vi "MH_T2 Read Acq Q_RawTimes.vi"() -> ()   [LabVIEW 2019]
uses:
  <userlib>/MultiHarp150/T2Lib/MH_T2QMessage.ctl
  <userlib>/MultiHarp150/T2Lib/MH_T2DeltaQMessage.ctl
  <vilib>/Analysis/NI_AALBase.lvlib
panel:
  out "valeur min":u64
  out "valeur max":u64
  out "Tableau":u64[][](array[numeric])
  out "Histogram: h(x)":i32[][](array[numeric])
  in  "Graphsamples":i32
  out "Graphe XY 2":T1(graph)
  in  "intervals":i32=10
  in  "Delta":bool
  in  "Graphe":bool
  out "Graphe XY":cluster{u64[], u64[]}[](graph)
  out "Photons":u64[][](array[numeric])
  out "taille(s)":i32[](array[numeric])
  out "Counters out":u32[](array[numeric])
  in  "TraceSize":u64
  in  "Bin size(ps)":u64
  in  "Tracelenght(s)":u64=16
  out "Done":bool
  out "TotalRec":i32
  out "TotalTime":u32
  in  "stop":bool
  out "sortie d'erreur":errorcluster caption="ErrorOut"
  out "RollOver":bool
  in  "Save Data":bool
  in  "StopCh":u32=2
  in  "StartCh":u32=1
  out "DeltaT":u32[](array[numeric])
  out "nActual":i32[](array[numeric])
  out "En Attente":i32[](array[numeric])
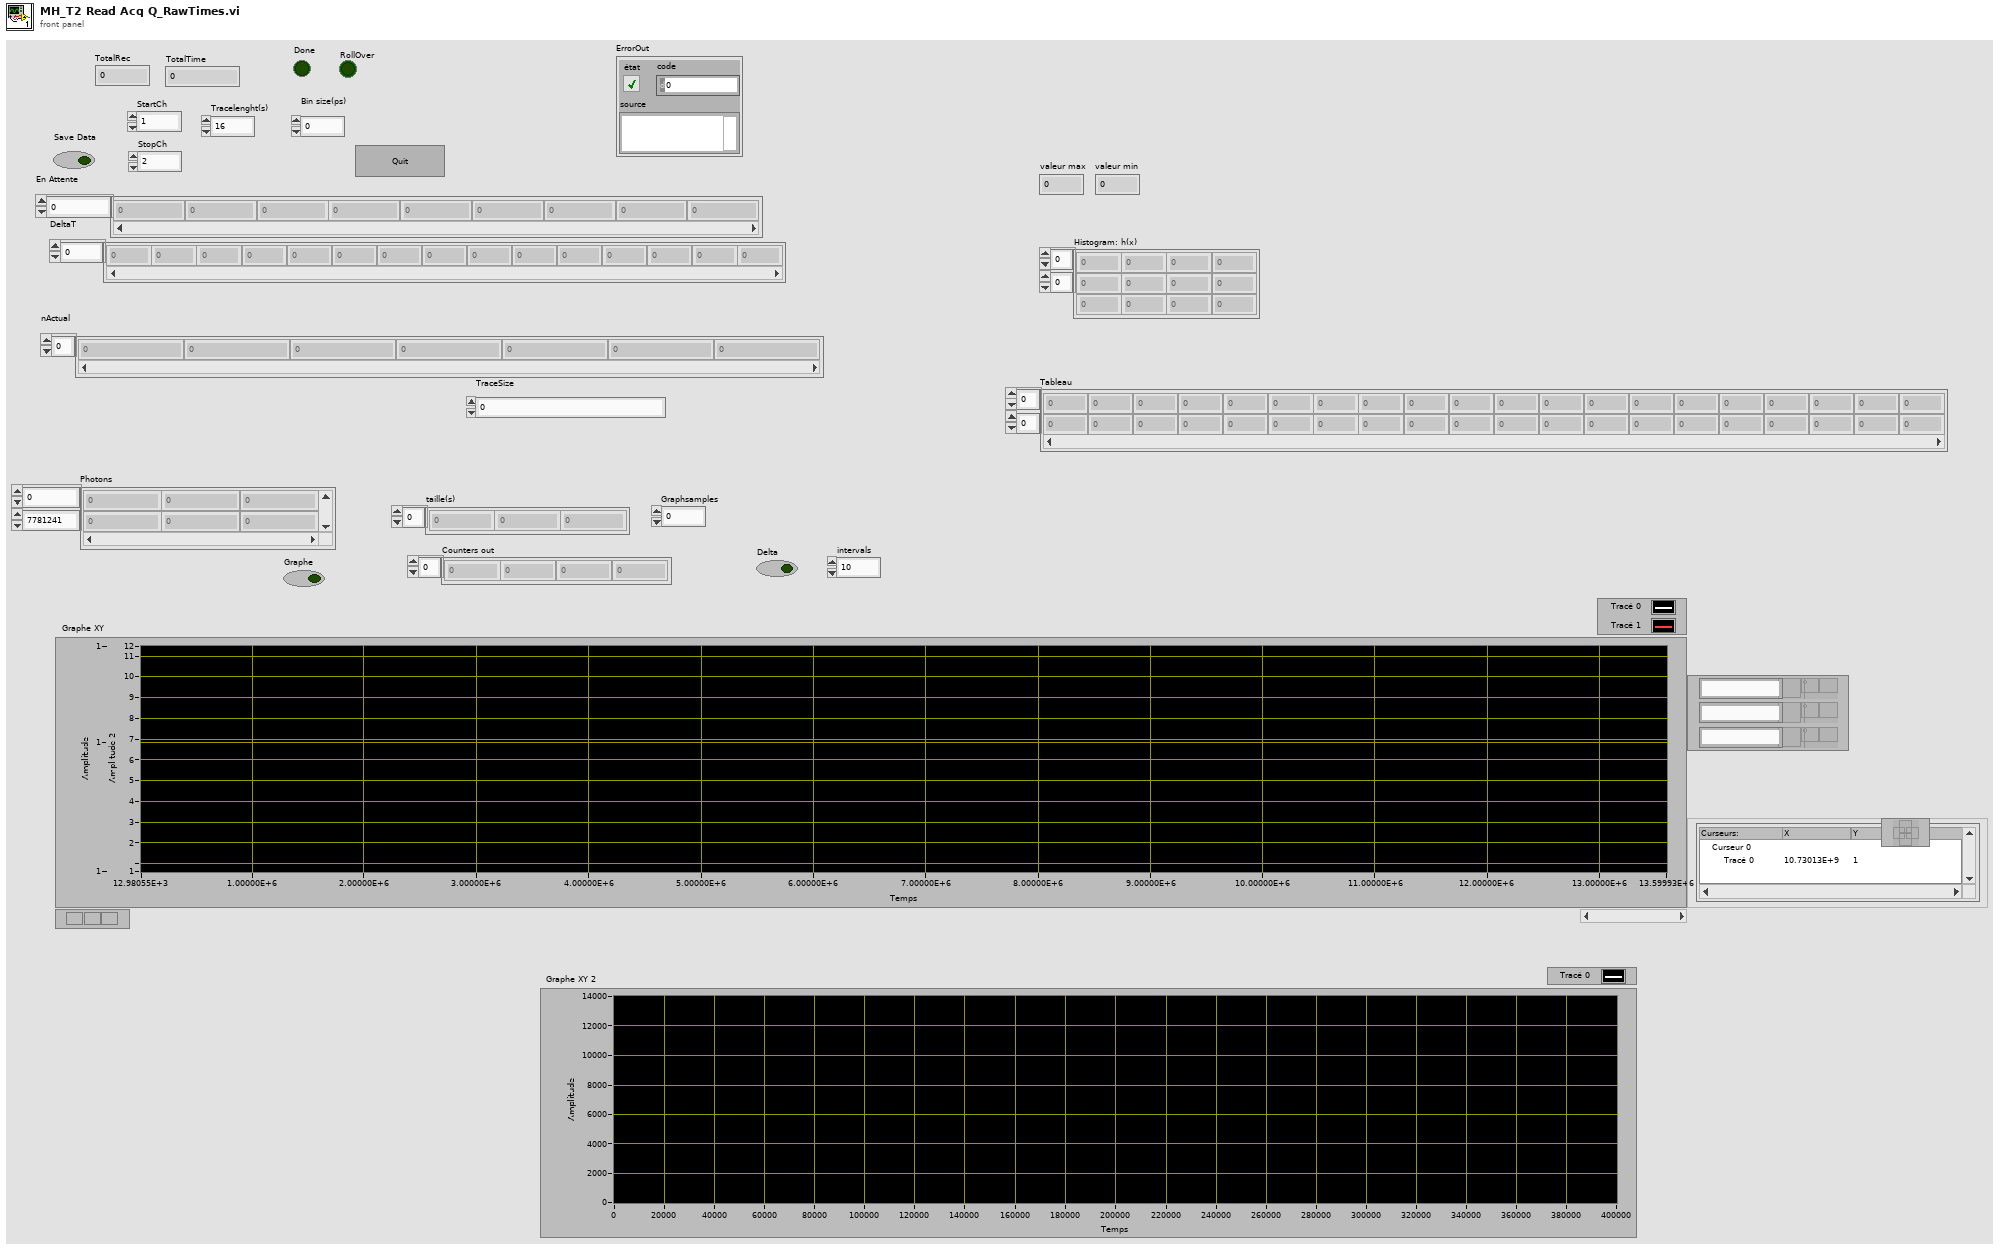
[diagram p1: front panel]
types:
  T1 = cluster{"X Values":dbl[], "Histogram: h(x)":i32[]}[]
  T2 = typedef "MH_T2DeltaQMessage.ctl" = cluster{"Message":string, "buffer":i32[], "Code":i32, "nactual":i32}
  T3 = typedef "MH_T2QMessage.ctl" = cluster{"Message":string, "buffer":u32[], "Code":i32, "nactual":i32}
  T4 = cluster{"X Values":dbl[], "Histogram: h(x)":i32[]}
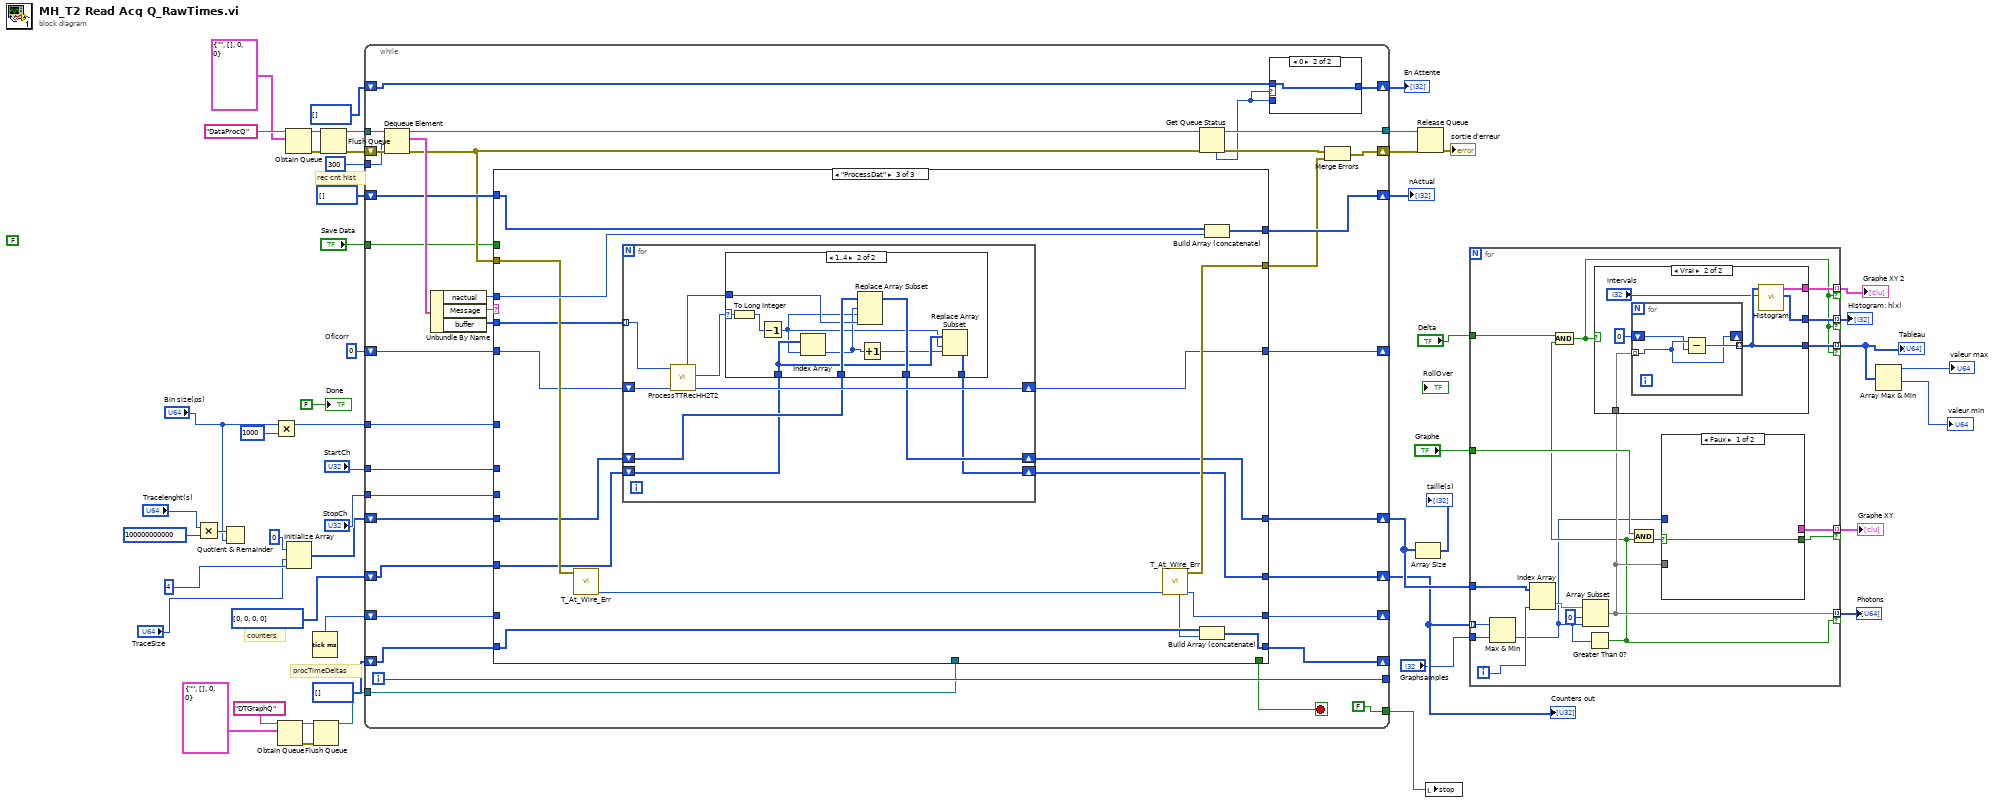
[diagram p0: block diagram]
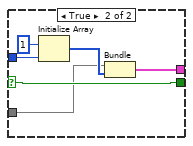
[diagram p3: hidden frame]
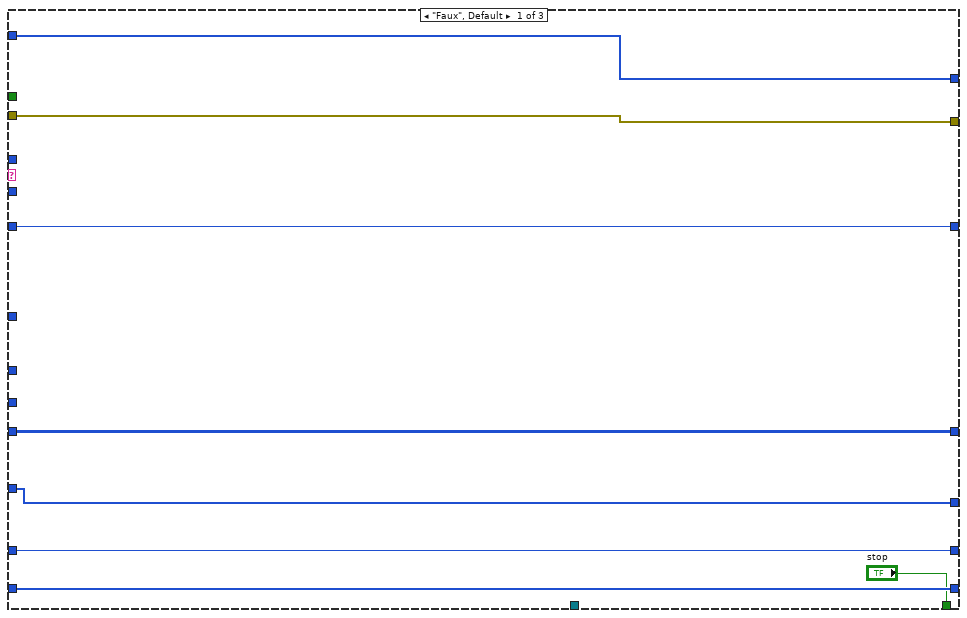
[diagram p4: hidden frame]
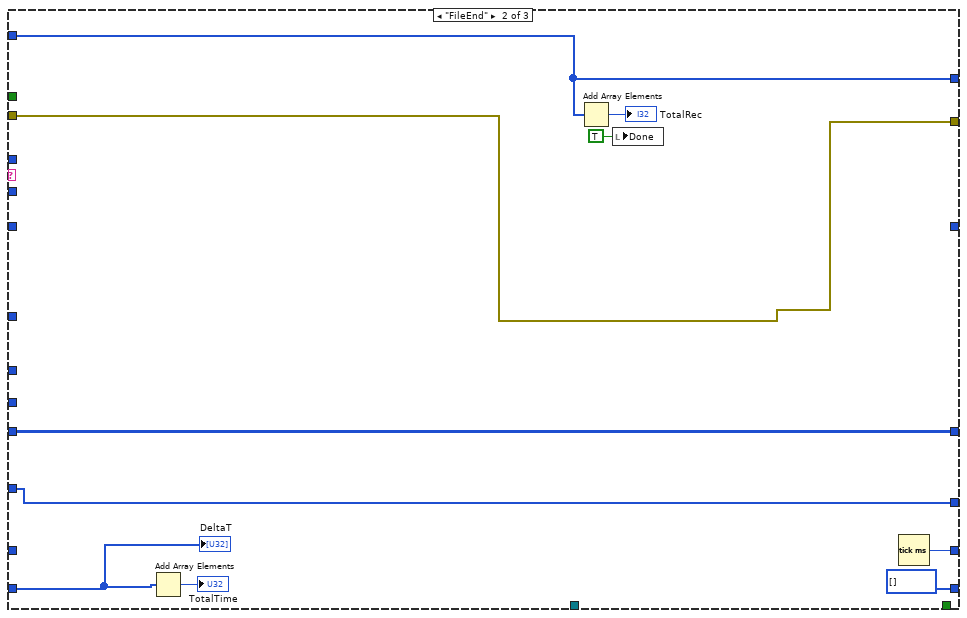
[diagram p5: hidden frame]
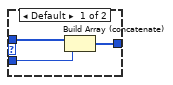
[diagram p7: hidden frame]
diagram:
  (unwired) FALSE
  w49 = u64 0  # Oflcorr
  # "counters"
  # "procTimeDeltas"
  # "rec cnt hist"
  n1 = Multiply(x="Tracelenght(s)", y=u64 100000000000) -> (x*y=w21:u64)
  n2 = Quotient & Remainder(x=w21, y="Bin size(ps)") -> ()  [unwired: 2 out]
  n3 = Multiply(x="Bin size(ps)", y=u64 1000) -> (x*y=w18:u64)
  n4 = Obtain Queue(name (unnamed)="DTGraphQ" ("nom (aucun)"), element data type=T2 {"Message"="", "buffer"=[], "Code"=0, "nactual"=0} ("ClassQueue")) -> (queue out=w27:refnum<queue>, error out=w28:errorcluster)  [unwired: 3 in, 1 out]
  n5 = Obtain Queue(name (unnamed)="DataProcQ" ("nom (aucun)"), element data type=T3 {"Message"="", "buffer"=[], "Code"=0, "nactual"=0} ("ClassQueue")) -> (queue out=w32:refnum<queue>, error out=w29:errorcluster)  [unwired: 3 in, 1 out]
  n6 = Initialize Array(u64 0 ("truetime"), "TraceSize", 4 ("taille de la dimension")) -> (w24:u64[][])
  n7 = Tick Count (ms)() -> (millisecond timer value=w45:u32)
  n8 = Flush Queue(queue=w27, error in (no error)=w28) -> (queue out=w34:refnum<queue>)  [unwired: 2 out]
  n9 = Flush Queue(queue=w32, error in (no error)=w29) -> (queue out=w31:refnum<queue>, error out=w30:errorcluster)  [unwired: 1 out]
  n10 = while {
    tunnel: w31 -> [w86]
    shift-right: [w67] -> w48
    shift-left: w30 -> [w87]
    shift-right: [w84] -> _
    shift-left: w49 -> [w85]
    tunnel: [w81] -> _
    tunnel: [w77] -> w47
    shift-right: [w75] -> _
    shift-left: w45 -> [w76]
    shift-right: [w73] -> _
    shift-left: u32[] [] ("DeltaT") -> [w74]
    shift-right: [w71] -> w42
    shift-left: i32[] [] ("DeltaT") -> [w72]
    shift-right: [w70] -> w46
    shift-left: i32[] [] ("DeltaT") -> [w69]
    tunnel: "Save Data" -> [w66]
    shift-right: [w63] -> w12
    shift-left: w24 -> [w65]
    tunnel: "StopCh" -> [w64]
    tunnel: 300 ("timeout en ms (-1)") -> [w62]
    tunnel: w34 -> [w60]
    tunnel: [FALSE] -> w26
    tunnel: "StartCh" -> [w55]
    tunnel: w18 -> [w54]
    shift-right: [w52] -> w11
    shift-left: i32[] [0, 0, 0, 0] ("DeltaT") -> [w53]
    i -> [w81]
    stop <- w58 stop-if-true
    n11 = Dequeue Element(queue=w86, timeout in ms (-1)=w62, error in (no error)=w87) -> (queue out=w79:refnum<queue>, element=w83:T3, error out=w68:errorcluster)  [unwired: 1 out]
    n12 = Unbundle By Name(w83) -> ("nactual"=w61:i32, "Message"=w80:string, "buffer"=w82:u32[])
    n13 = case shown="\"ProcessDat\"" w80 {
      tunnel: w85 -> [w95 _ w111]
      tunnel: [w95 _ w110] -> w84
      tunnel: w82 -> [_ _ w112]
      tunnel: w76 -> [w94 _ _]
      tunnel: [w93 u32[] [] ("DeltaT") w115] -> w73
      tunnel: [w94 w104 w116] -> w75
      tunnel: w74 -> [w93 w102 w114]
      tunnel: w72 -> [w92 w100 w121]
      tunnel: [w92 w100 w122] -> w71
      tunnel: w68 -> [w90 w97 w119]
      tunnel: w66 -> [_ _ _]
      tunnel: w65 -> [w91 w105 w109]
      tunnel: w64 -> [_ _ _]
      tunnel: [w91 w105 w108] -> w63
      tunnel: w61 -> [_ _ w120]
      tunnel: w60 -> [_ _ _]
      tunnel: [w90 w97 w118] -> w59
      tunnel: ["stop" _ _] -> w58
      tunnel: w55 -> [_ _ _]
      tunnel: w54 -> [_ _ _]
      tunnel: w53 -> [w88 w96 w107]
      tunnel: [w88 w96 w106] -> w52
      frame "Faux", Default {
      }
      frame "FileEnd" {
        n14 = Add Array Elements(numeric array=w102) -> (sum=→"TotalTime":u32)
        n15 = Add Array Elements(numeric array=w100) -> (sum=→"TotalRec":i32)
        n16 = local write "Done"(TRUE ("Done")) -> ()
        n17 = Tick Count (ms)() -> (millisecond timer value=w104:u32)
        "DeltaT" <- w102
      }
      frame "ProcessDat" {
        n18 = call <userlib>:"T_At_Wire_Err.vi"("error in (no error)"=w119) -> ("Clock(ms)"=w117:u32)  [unwired: 8 in, 2 out]
        n19 = for {
          tunnel: w112 -> [w131] mode=indexing
          shift-right: [w129] -> w110
          shift-left: w111 -> [w130]
          shift-right: [w125] -> w108
          shift-left: w109 -> [w126]
          shift-right: [w123] -> w106
          shift-left: w107 -> [w124]
          n20 = call <userlib>:"ProcessTTRecHH2T2.vi"("oflcorr_in"=w130, "rawbits"=w131) -> ("oflcorr_out"=w129:u64, "channel"=w128:u32, "truetime"=w127:u64)  [unwired: 4 in, 3 out]
          n21 = case shown="1..4" w128 {
            selector: w128 -> [_ w137]
            tunnel: w127 -> [_ w141]
            tunnel: w126 -> [w133 w143]
            tunnel: [w133 w142] -> w125
            tunnel: w124 -> [w132 w139]
            tunnel: [w132 w135] -> w123
            frame 0, Default {
            }
            frame 1..4 {
              n22 = To Long Integer(number=w137) -> (32bit integer=w136:i32)
              n23 = Decrement(x=w136) -> (x-1=w134:i32)
              n24 = Index Array(array=w139, index=w134) -> (element=w140:i32)
              n25 = Replace Array Subset(array=w143, new element=w141, index (row)=w140, index (col)=w134) -> (w142:u64[][])
              n26 = Increment(x=w140) -> (x+1=w138:i32)
              n27 = Replace Array Subset(array=w139, new element=w138, index=w134) -> (w135:i32[])
            }
          }
        }
        n28 = call <userlib>:"T_At_Wire_Err.vi"("InitClock(ms)"=w117) -> ("Clock(ms)"=w116:u32, "error out"=w118:errorcluster, "Delta(ms)"=w113:u32)  [unwired: 8 in]
        n29 = Build Array (concatenate)(w114, w113) -> (w115:u32[])
        n30 = Build Array (concatenate)(w121, w120) -> (w122:i32[])
      }
    }
    n31 = Get Queue Status(queue=w79, error in (no error)=w68) -> (queue out=w77:refnum<queue>, error out=w78:errorcluster, # elements in queue=w56:i32)  [unwired: 1 in, 5 out]
    n32 = case shown="0" w56 {
      tunnel: w56 -> [w146 _]
      tunnel: [w145 w147] -> w70
      tunnel: w69 -> [w144 w147]
      frame Default {
        n33 = Build Array (concatenate)(w144, w146) -> (w145:i32[])
      }
      frame 0 {
      }
    }
    n34 = Merge Errors(w78, w59) -> (w67:errorcluster)
  }
  "En Attente" <- w46
  "nActual" <- w42
  "Counters out" <- w11
  n35 = Array Size(array=w12) -> (size(s)=→"taille(s)":i32[])
  n36 = Release Queue(queue=w47, error in (no error)=w48) -> (error out=→"sortie d'erreur":errorcluster)  [unwired: 1 in, 2 out]
  n37 = local write "stop"(w26) -> ()
  n38 = for {
    tunnel: w12 -> [w165]
    tunnel: w11 -> [w152] mode=indexing
    tunnel: [w157] -> w10 mode=indexing if=w155
    tunnel: [w161] -> w8 mode=indexing if=w160
    tunnel: "Graphe" -> [w158]
    tunnel: "Delta" -> [w156]
    tunnel: [w154] -> w3 mode=indexing if=w148
    tunnel: [w153] -> w6 mode=indexing if=w148
    tunnel: "Graphsamples" -> [w151]
    tunnel: [w149] -> w4 mode=indexing if=w148
    i -> [w164]
    n39 = Max & Min(x=w152, y=w151) -> (min(x,y)=w150:i32)  [unwired: 1 out]
    n40 = Index Array(array=w165, index (col)=w164) -> (element=w163:u64[])  [unwired: 1 in]
    n41 = Array Subset(array=w163, index=0 ("indice"), length=w150) -> (w157:u64[])
    n42 = Greater Than 0?(x=w150) -> (x > 0?=w155:bool)
    n43 = And(x=w156, y=w155) -> (x .and. y?=w148:bool)
    n44 = case shown="Vrai" w148 {
      tunnel: w157 -> [_ w171]
      tunnel: [_ w169] -> w154
      tunnel: [_ w167] -> w153
      tunnel: [_ w166] -> w149
      frame False {
      }
      frame True {
        n45 = for {
          tunnel: w171 -> [w173] mode=indexing
          shift-right: [w173] -> _
          shift-left: u64 0 ("truetime") -> [w172]
          tunnel: [w174] -> w169 mode=indexing
          n46 = Subtract(x=w173, y=w172) -> (x-y=w174:u64)
        }
        n47 = call <vilib>:"Histogram.vi"("intervals"="intervals", "X"=w169) -> ("Histogram: h(x)"=w166:i32[], "Histogram Graph"=w167:T4)  [unwired: 6 in, 2 out]
      }
    }
    n48 = And(x=w158, y=w155) -> (x .and. y?=w159:bool)
    n49 = case shown="Faux" w159 {
      selector: w159 -> [w175 w178]
      tunnel: w157 -> [_ w176]
      tunnel: w150 -> [_ w181]
      tunnel: [_ w179] -> w161
      tunnel: [w175 w178] -> w160
      frame False {
      }
      frame True {
        n50 = Initialize Array(u64 1 ("élément"), w181) -> (w177:u64[])
        n51 = Bundle(w176, w177) -> (w179:cluster{u64[], u64[]})  [unwired: 1 in]
      }
    }
  }
  "Photons" <- w10
  "Graphe XY" <- w8
  "Graphe XY 2" <- w6
  "Histogram: h(x)" <- w4
  "Tableau" <- w3
  n52 = Array Max & Min(array=w3) -> (max value=→"valeur max":u64, min value=→"valeur min":u64)  [unwired: 2 out]
  "Done" <- FALSE
